vi "Trasparentar.vi"(10 "Background Color":u32(colorbox)=16777215, 11 "24-bit pixmap":u32[][](array[numeric]) format="%x") -> (3 "Mask":u8[](array[numeric]))   [LabVIEW 2017]
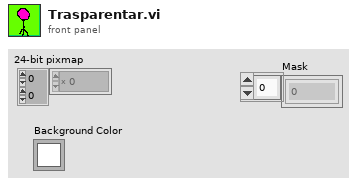
[diagram p1: front panel]
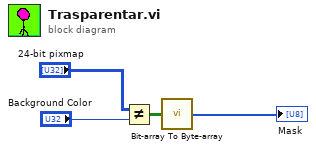
[diagram p0: block diagram]
diagram:
  n1 = Not Equal?(x="24-bit pixmap", y="Background Color") -> (x != y?=w3:bool[][])
  n2 = call <vilib>:"Bit-array To Byte-array.vi"("bit array"=w3) -> ("byte array"=→"Mask":u8[])
